vi "Get Connector Pane State.vi"(8 "error in (no error)":errorcluster, 11 "PPL in":refnum<class "NI_AB_API_PPL.lvclass">) -> (0 "error out":errorcluster, 2 "callers adapt?":bool, 3 "PPL out":refnum<class "NI_AB_API_PPL.lvclass">)   [LabVIEW 2020, in "NI_AB_API_PPL.lvclass"]
uses:
  <vilib>/AppBuilder/AB_API/PPL/NI_AB_API_PPL.lvclass
  e:/builds/penguin/labview/branches/2020/dev/dist/vi.lib/AppBuilder/AB_API/Build/NI_AB_API_Build.lvclass
  <vilib>/AppBuilder/AB_Classes/PackedLib/AB_PackedLibrary.lvclass
  <vilib>/AppBuilder/AB_API/PPL/NI_AB_API_PPL.lvclass/NI_AB_API_PPL.ctl
  <vilib>/AppBuilder/AB_API/Build/NI_AB_API_Build.lvclass
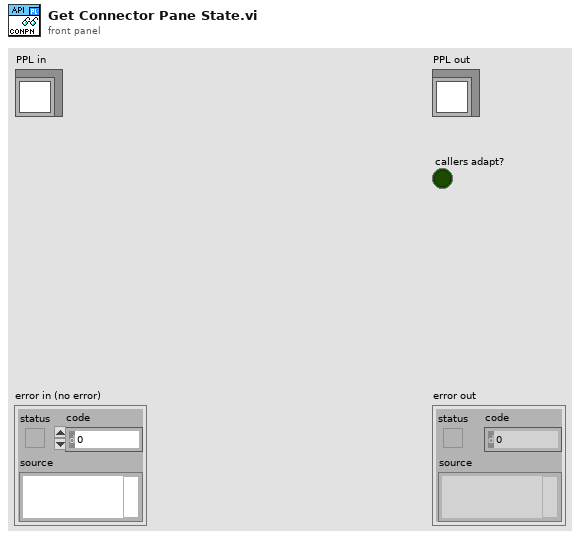
[diagram p1: front panel]
types:
  T1 = typedef "AB_PackedLibrary.ctl" = cluster{"callersAdapt":bool, "showWarnings":bool, "verifyConnpane":bool, "eng_sourceLibrary":string, "eng_packedLib_inMemory":bool}
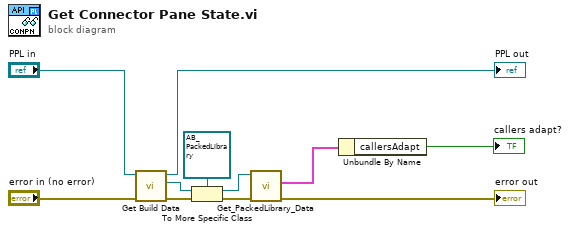
[diagram p0: block diagram]
diagram:
  n1 = call <vilib>:"Get Build Data.vi"("error in (no error)"="error in (no error)", "NI_AB_API_Build in"="PPL in") -> ("error out"=w3:errorcluster, "AB_Build.lvclass"=w4:refnum<class "AB_Build.lvclass">, "NI_AB_API_Build out"=→"PPL out":refnum<class "NI_AB_API_PPL.lvclass">)  [unwired: 7 in]
  n2 = To More Specific Class(target class=refnum<class "AB_PackedLibrary.lvclass"> refnum ("AB_PackedLibrary.lvclass"), reference=w4, error in=w3) -> (specific class reference=w5:refnum<class "AB_PackedLibrary.lvclass">, error out=w2:errorcluster)
  n3 = call <vilib>:"Get_PackedLibrary_Data.vi"("error in (no error)"=w2, "Class in"=w5) -> ("error out"=→"error out":errorcluster, "data"=w8:T1)  [unwired: 7 in, 1 out]
  n4 = Unbundle By Name(w8) -> ("callersAdapt"=→"callers adapt?":bool)
